vi "Configure AIN (depreciated).vi"() -> ()   [LabVIEW 2021]
panel:
  in  "AIN Range":u16(ring)=2 items=["LJ_rgBIP20V", "LJ_rgBIP10V", "LJ_rgBIP5V", "LJ_rgBIP4V", "LJ_rgBIP2P5V", "LJ_rgBIP2V", "LJ_rgBIP1P25V", "LJ_rgBIP1V", "LJ_rgBIPP625V", "LJ_rgUNI20V", "LJ_rgUNI10V", "LJ_rgUNI5V", "LJ_rgUNI4V", "LJ_rgUNI2P5V", "LJ_rgUNI2V", "LJ_rgUNI1P25V", "LJ_rgUNI1V", "LJ_rgUNIP625V"]
  in  "Do Not Do Go()":bool
  in  "ChannelNum, Range Constant":i32[][](array[numeric])
  in  "Binary":bool
  in  "SettlingFactor":i32
  in  "Handle In":i32
  in  "error in":errorcluster
  out "error out":errorcluster
  out "Handle Out":i32
  in  "Resolution":i32=12
  # "If true, requests will be added but not executed.\nSaves time if this VI is going to be following by\nanother VI which will do the Go(), but you do not\nget any errorcodes thrown by these config requests.\nUsually, this can be left FALSE as this function is only\ncalled once at the beginning of a program."
  # "Used to get range constant strings"
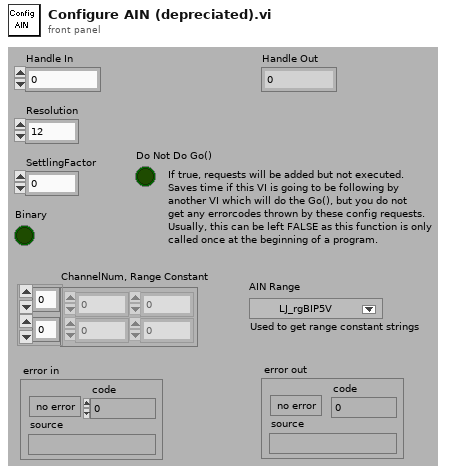
[diagram p1: front panel]
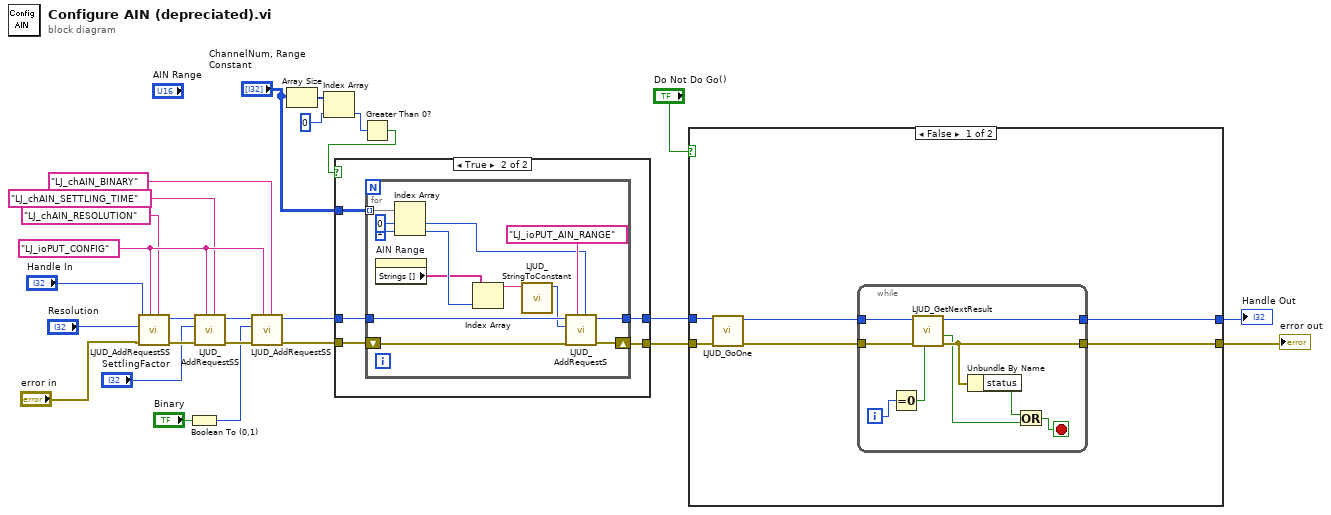
[diagram p0: block diagram]
diagram:
  w19 = "LJ_ioPUT_CONFIG" ("IOType")
  n1 = call "LJUD_AddRequestSS.vi"("Channel"="LJ_chAIN_RESOLUTION" ("IOType"), "IOType"=w19, "error in"="error in", "Value"="Resolution", "Handle In"="Handle In") -> ("error out"=w21:errorcluster, "Handle Out"=w23:i32)  [unwired: 5 in]
  n2 = Boolean To (0,1)(Boolean="Binary") -> (0, 1=w13:i16)
  n3 = call "LJUD_AddRequestSS.vi"("Channel"="LJ_chAIN_SETTLING_TIME" ("IOType"), "IOType"=w19, "error in"=w21, "Value"="SettlingFactor", "Handle In"=w23) -> ("error out"=w20:errorcluster, "Handle Out"=w22:i32)  [unwired: 5 in]
  n4 = call "LJUD_AddRequestSS.vi"("Channel"="LJ_chAIN_BINARY" ("IOType"), "IOType"=w19, "error in"=w20, "Value"=w13, "Handle In"=w22) -> ("error out"=w9:errorcluster, "Handle Out"=w10:i32)  [unwired: 5 in]
  n5 = Array Size(array="ChannelNum, Range Constant") -> (size(s)=w12:i32[])
  n6 = Index Array(array=w12, index=0 ("Index")) -> (element=w1:i32)
  n7 = Greater Than 0?(x=w1) -> (x > 0?=w2:bool)
  n8 = case shown="True" w2 {
    tunnel: w10 -> [w28 w33]
    tunnel: w9 -> [w27 w32]
    tunnel: "ChannelNum, Range Constant" -> [_ w31]
    tunnel: [w28 w30] -> w6
    tunnel: [w27 w29] -> w5
    frame False {
    }
    frame True {
      n9 = for {
        tunnel: w33 -> [w46]
        shift-right: [w43] -> w29
        shift-left: w32 -> [w44]
        tunnel: w31 -> [w42] mode=indexing
        tunnel: [w39] -> w30
        n10 = property on="AIN Range" class="Ring (strict)"() -> ("Strings []"=w34:string[])  [unwired: 2 in, 2 out]
        n11 = Index Array(array=w42, index #1=0 ("Index"), index #2=1 ("Index")) -> (element #1=w36:i32, element #2=w37:i32)
        n12 = Index Array(array=w34, index=w37) -> (element=w35:string)
        n13 = call "LJUD_StringToConstant.vi"("String"=w35) -> ("Constant Number"=w38:i32)  [unwired: 9 in, 1 out]
        n14 = call "LJUD_AddRequestS.vi"("Channel"=w36, "IOType"="LJ_ioPUT_AIN_RANGE", "error in"=w44, "Value"=w38, "Handle In"=w46) -> ("error out"=w43:errorcluster, "Handle Out"=w39:i32)  [unwired: 5 in]
      }
    }
  }
  n15 = case shown="False" "Do Not Do Go()" {
    tunnel: w6 -> [w52 w63]
    tunnel: w5 -> [w51 w62]
    tunnel: [w48 w63] -> w4
    tunnel: [w47 w62] -> w3
    frame False {
      n16 = call "LJUD_GoOne.vi"("error in"=w51, "Handle In"=w52) -> ("error out"=w50:errorcluster, "Handle Out"=w49:i32)  [unwired: 8 in]
      n17 = while {
        tunnel: w50 -> [w59]
        tunnel: w49 -> [w58]
        tunnel: [w57] -> w47
        tunnel: [w55] -> w48
        i -> [w54]
        stop <- w61 stop-if-true
        n18 = Equal To 0?(x=w54) -> (x = 0?=w60:bool)
        n19 = call "LJUD_GetNextResult.vi"("GetFirst"=w60, "error in"=w59, "Handle In"=w58) -> ("error out"=w57:errorcluster, "LJE_NO_MORE_DATA_AVAILABLE"=w53:bool, "Handle Out"=w55:i32)  [unwired: 3 in, 3 out]
        n20 = Unbundle By Name(w57) -> ("status"=w56:bool)
        n21 = Or(x=w56, y=w53) -> (x .or. y?=w61:bool)
      }
    }
    frame True {
    }
  }
  "Handle Out" <- w4
  "error out" <- w3
